vi "DispList _ Initialize List.vi"(8 "error in":errorcluster caption="错误输入", 11 "ref":refnum<vi>) -> (0 "error out":errorcluster caption="错误输出", 3 "ref":refnum<vi>)   [LabVIEW 2016]
uses:
  <vilib>/Utility/miscctls.llb/LVRowAndColumnTypeDef.ctl
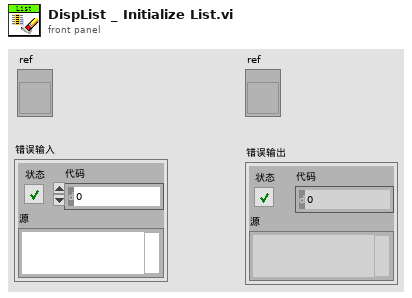
[diagram p1: front panel]
types:
  T1 = typedef "LVRowAndColumnTypeDef.ctl" = cluster{"Row":i32, "Column":i32}
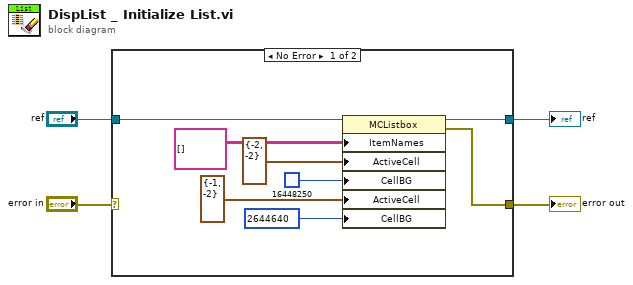
[diagram p0: block diagram]
diagram:
  n1 = case shown="No Error" "error in" {
    selector: "error in" -> [_ w14]
    tunnel: [w5 w14] -> w3
    tunnel: "ref" -> [w7 w13]
    tunnel: [w6 w13] -> w1
    frame No Error {
      n2 = property class="MCListbox"(reference=w7, "ItemNames"=string[][] [] ("项名"), "ActiveCell"=T1 {"Row"=-2, "Column"=-2} ("活动单元格:活动单元格"), "CellBG"=u32 16448250, "ActiveCell"=T1 {"Row"=-1, "Column"=-2} ("活动单元格:活动单元格"), "CellBG"=u32 2644640 ("活动单元格:单元格背景色")) -> (reference out=w6:refnum<vi>, error out=w5:errorcluster)  [unwired: 1 in]
    }
    frame Error {
    }
  }
  "error out" <- w3
  "ref" <- w1
